vi "RichToFlatcif_manager_QueryPluginTypesResponse.vi"(5 "OutputClusterType":T1, 11 "InputCluster":T5) -> (3 "OutputCluster":T1)   [LabVIEW 2021, in "CIF_Manager_server.lvlib"]
uses:
  CIF_Manager_server.lvlib
  cif_manager_QueryPluginTypesResponse.ctl
  cif_manager_PluginType.ctl
  cif_common_ShortVersion.ctl
  cif_management_common_PluginMetadata.ctl
  cif_manager_QueryPluginTypesResponse_Flat.ctl
  cif_manager_PluginType_Flat.ctl
  cif_common_ShortVersion_Flat.ctl
  cif_management_common_PluginMetadata_Flat.ctl
  RichToFlatcif_common_ShortVersion.vi
  RichToFlatcif_management_common_PluginMetadata.vi
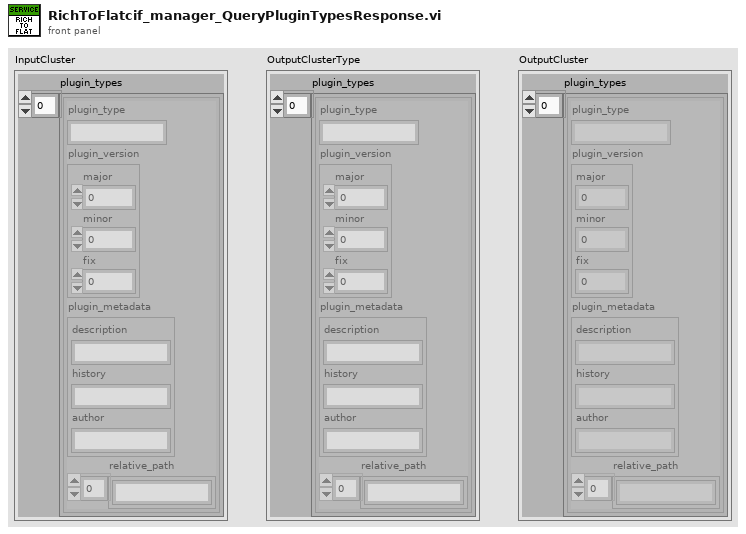
[diagram p1: front panel]
types:
  T1 = typedef "CIF_Manager_server.lvlib/cif_manager_QueryPluginTypesResponse_Flat.ctl" = cluster{"plugin_types":T2[]}
  T2 = typedef "CIF_Manager_server.lvlib/cif_manager_PluginType_Flat.ctl" = cluster{"plugin_type":string, "plugin_version":T3, "plugin_metadata":T4, "relative_path":string[]}
  T3 = typedef "CIF_Manager_server.lvlib/cif_common_ShortVersion_Flat.ctl" = cluster{"major":u32, "minor":u32, "fix":u32}
  T4 = typedef "CIF_Manager_server.lvlib/cif_management_common_PluginMetadata_Flat.ctl" = cluster{"description":string, "history":string, "author":string}
  T5 = typedef "CIF_Manager_server.lvlib/cif_manager_QueryPluginTypesResponse.ctl" = cluster{"plugin_types":T6[]}
  T6 = typedef "CIF_Manager_server.lvlib/cif_manager_PluginType.ctl" = cluster{"plugin_type":string, "plugin_version":T7, "plugin_metadata":T8, "relative_path":string[]}
  T7 = typedef "CIF_Manager_server.lvlib/cif_common_ShortVersion.ctl" = cluster{"major":u32, "minor":u32, "fix":u32}
  T8 = typedef "CIF_Manager_server.lvlib/cif_management_common_PluginMetadata.ctl" = cluster{"description":string, "history":string, "author":string}
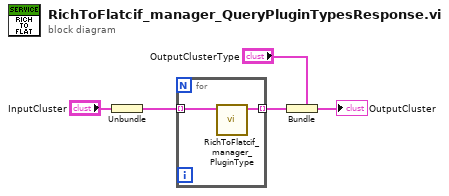
[diagram p0: block diagram]
diagram:
  n1 = Unbundle "Unbundle"("InputCluster") -> ("plugin_types"=w2:T6[])
  n2 = for {
    tunnel: w2 -> [w7] mode=indexing
    tunnel: [w6] -> w1 mode=indexing
    n3 = call "RichToFlatcif_manager_PluginType.vi"("InputCluster"=w7) -> ("OutputCluster"=w6:T2)  [unwired: 10 in]
  }
  n4 = Bundle "Bundle"(cluster="OutputClusterType", "plugin_types"=w1) -> (→"OutputCluster":T1)
